vi "Theta 0.vi"(10 "theta_6":dbl, 11 "6R Type 1 Serial Arm Class in":refnum<class "NI_Robotics_6R Type 1 Serial Arm Class.lvclass">) -> (0 "Valid?":bool, 1 "XYZ_6":dbl[](array[numeric]), 2 "theta_0 array":dbl[](array[numeric]), 3 "6R Type 1 Serial Arm Class out":refnum<class "NI_Robotics_6R Type 1 Serial Arm Class.lvclass">)   [LabVIEW 2017, in "NI_Robotics_6R Type 1 Serial Arm Class.lvclass"]
uses:
  <vilib>/robotics/Kinematics/Analytical/6R/Type 1/NI_Robotics_6R Type 1 Serial Arm Class.lvclass
  c:/Program Files (x86)/National Instruments/LabVIEW 2017/vi.lib/robotics/Kinematics/Analytical/Generic/NI_Robotics_Analytical Serial Arm Class.lvclass
  <vilib>/robotics/Kinematics/Link/NI_Robotics_Link.lvclass/NI_Robotics_Link.ctl
  <vilib>/robotics/Kinematics/Analytical/6R/Type 1/NI_Robotics_6R Type 1 Serial Arm Class.lvclass/NI_Robotics_6R Type 1 Serial Arm Class.ctl
  <vilib>/robotics/Kinematics/Link/Get Kinematic Parameters.vi
  <vilib>/robotics/Kinematics/Analytical/Generic/NI_Robotics_Analytical Serial Arm Class.lvclass
  c:/Program Files (x86)/National Instruments/LabVIEW 2017/vi.lib/robotics/Kinematics/Robot/NI_Robotics_Serial Robot Arm.lvclass
  <vilib>/robotics/Kinematics/Analytical/Generic/Accessors/Read alpha_n0.vi
  <vilib>/robotics/Kinematics/Robot/Get Links.vi
  <vilib>/robotics/Kinematics/Analytical/NI_Robotics_AnalyticKinematics.lvlib
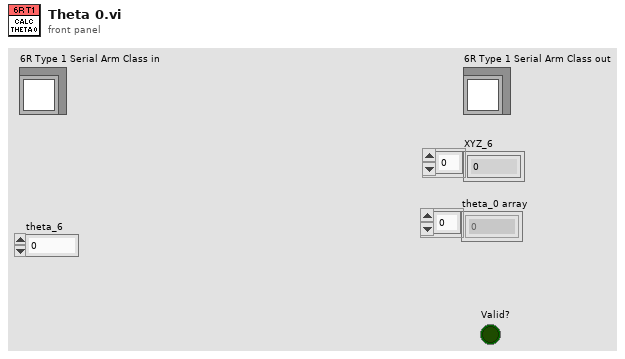
[diagram p1: front panel]
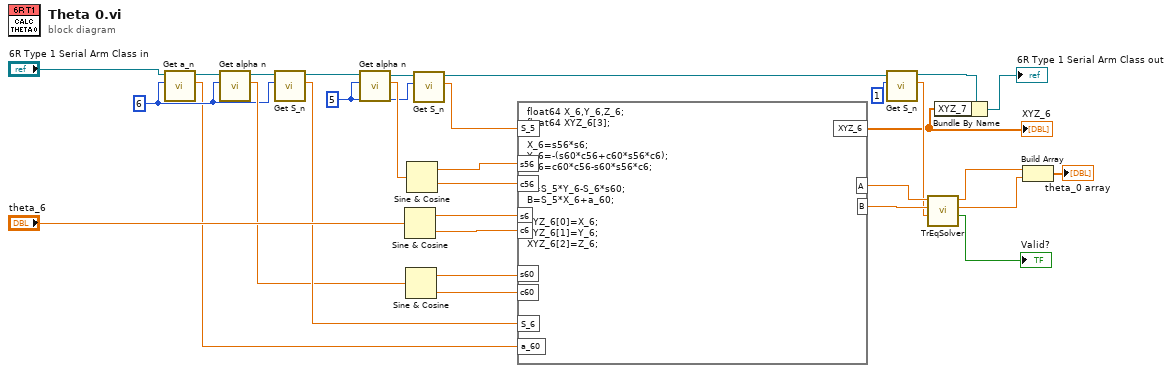
[diagram p0: block diagram]
diagram:
  w5 = 6 ("n")
  w22 = 5 ("n")
  n1 = call <vilib>:"Get a_n.vi"("n"=w5, "Analytical Serial Arm Class in"="6R Type 1 Serial Arm Class in") -> ("a_n"=w4:dbl, "Analytical Serial Arm Class out"=w7:refnum<class "NI_Robotics_6R Type 1 Serial Arm Class.lvclass">)  [unwired: 8 in]
  n2 = call <vilib>:"Get alpha n.vi"("n"=w5, "Analytical Serial Arm Class in"=w7) -> ("alpha n"=w8:dbl, "Analytical Serial Arm Class out"=w11:refnum<class "NI_Robotics_6R Type 1 Serial Arm Class.lvclass">)  [unwired: 8 in]
  n3 = call <vilib>:"Get S_n.vi"("n"=w5, "Analytical Serial Arm Class in"=w11) -> ("S_n"=w9:dbl, "Analytical Serial Arm Class out"=w10:refnum<class "NI_Robotics_6R Type 1 Serial Arm Class.lvclass">)  [unwired: 8 in]
  n4 = call <vilib>:"Get alpha n.vi"("n"=w22, "Analytical Serial Arm Class in"=w10) -> ("alpha n"=w31:dbl, "Analytical Serial Arm Class out"=w23:refnum<class "NI_Robotics_6R Type 1 Serial Arm Class.lvclass">)  [unwired: 8 in]
  n5 = Sine & Cosine(0:"theta_6") -> (1:w27:dbl, 2:w26:dbl)
  n6 = Sine & Cosine(0:w8) -> (1:w25:dbl, 2:w24:dbl)
  n7 = Sine & Cosine(0:w31) -> (1:w29:dbl, 2:w28:dbl)
  n8 = call <vilib>:"Get S_n.vi"("n"=w22, "Analytical Serial Arm Class in"=w23) -> ("S_n"=w21:dbl, "Analytical Serial Arm Class out"=w20:refnum<class "NI_Robotics_6R Type 1 Serial Arm Class.lvclass">)  [unwired: 8 in]
  n9 = formula code="float64 X_6,Y_6,Z_6;\nfloat64 XYZ_6[3];\n\nX_6=s56*s6;\nY_6=-(s60*c56+c60*s56*c6);\nZ_6=c60*c56-s60*s56*c6;\n\nA=S_5*Y_6-S_6*s60;\nB=S_5*X_6+a_60;\n\nXYZ_6[0]=X_6;\nXYZ_6[1]=Y_6;\nXYZ_6[2]=Z_6;"("s56"=w29, "c56"=w28, "s6"=w27, "c6"=w26, "s60"=w25, "c60"=w24, "S_5"=w21, "S_6"=w9, "a_60"=w4) -> ("A"=w18:dbl, "B"=w17:dbl, "XYZ_6"=w14:dbl[])
  "XYZ_6" <- w14
  n10 = call <vilib>:"Get S_n.vi"("n"=1, "Analytical Serial Arm Class in"=w20) -> ("S_n"=w16:dbl, "Analytical Serial Arm Class out"=w13:refnum<class "NI_Robotics_6R Type 1 Serial Arm Class.lvclass">)  [unwired: 8 in]
  n11 = call <vilib>:"TrEqSolver.vi"("D"=w16, "B"=w17, "A"=w18) -> ("Solution Exists"=→"Valid?":bool, "angle 2"=w2:dbl, "angle 1"=w3:dbl)  [unwired: 6 in]
  n12 = Bundle By Name(cluster=w13, "XYZ_7"=w14) -> (→"6R Type 1 Serial Arm Class out":refnum<class "NI_Robotics_6R Type 1 Serial Arm Class.lvclass">)
  n13 = Build Array(w3, w2) -> (→"theta_0 array":dbl[])
